vi "Get minimum separation within sphere.vi"(0 "Triangles to test":T2[](array[typedef]), 1 "Query triangles":T2[](array[typedef]), 2 "Octree for query triangles":T3[](array[typedef]), 3 "Sphere of interest":T1) -> (6 "Minimum separation vector\n(from all test triangles)":sgl[](array[numeric]), 7 "Minimum separation":sgl, 8 "Indices of possible triangles":i32[](array[numeric]))   [LabVIEW 2017]
doc: "This VI returns all the collision points between the test triangle and the query triangles, as well as the minimum separation vector and distance in the case of no collision."
uses:
  Typedefs/Triangle.ctl
  Typedefs/TreeNodeBox.ctl
  Typedefs/Quad.ctl
  Typedefs/Quadplane enum.ctl
  Typedefs/Sphere.ctl
panel:
  # "PN 13/03/2015"
  # "Vertices"
  # "Edges"
  # "Unit normal"
  # "Edge unit normals"
  # "Vertices"
  # "Edges"
  # "Unit normal"
  # "Plane ident."
  # "Vertices"
  # "Edges"
  # "Unit normal"
  # "Plane ident."
  # "Vertices"
  # "Edges"
  # "Unit normal"
  # "Plane ident."
  # "Vertices"
  # "Edges"
  # "Unit normal"
  # "Plane ident."
  # "Vertices"
  # "Edges"
  # "Unit normal"
  # "Plane ident."
  # "Vertices"
  # "Edges"
  # "Unit normal"
  # "Plane ident."
  # "Vertices"
  # "Edges"
  # "Unit normal"
  # "Edge unit normals"
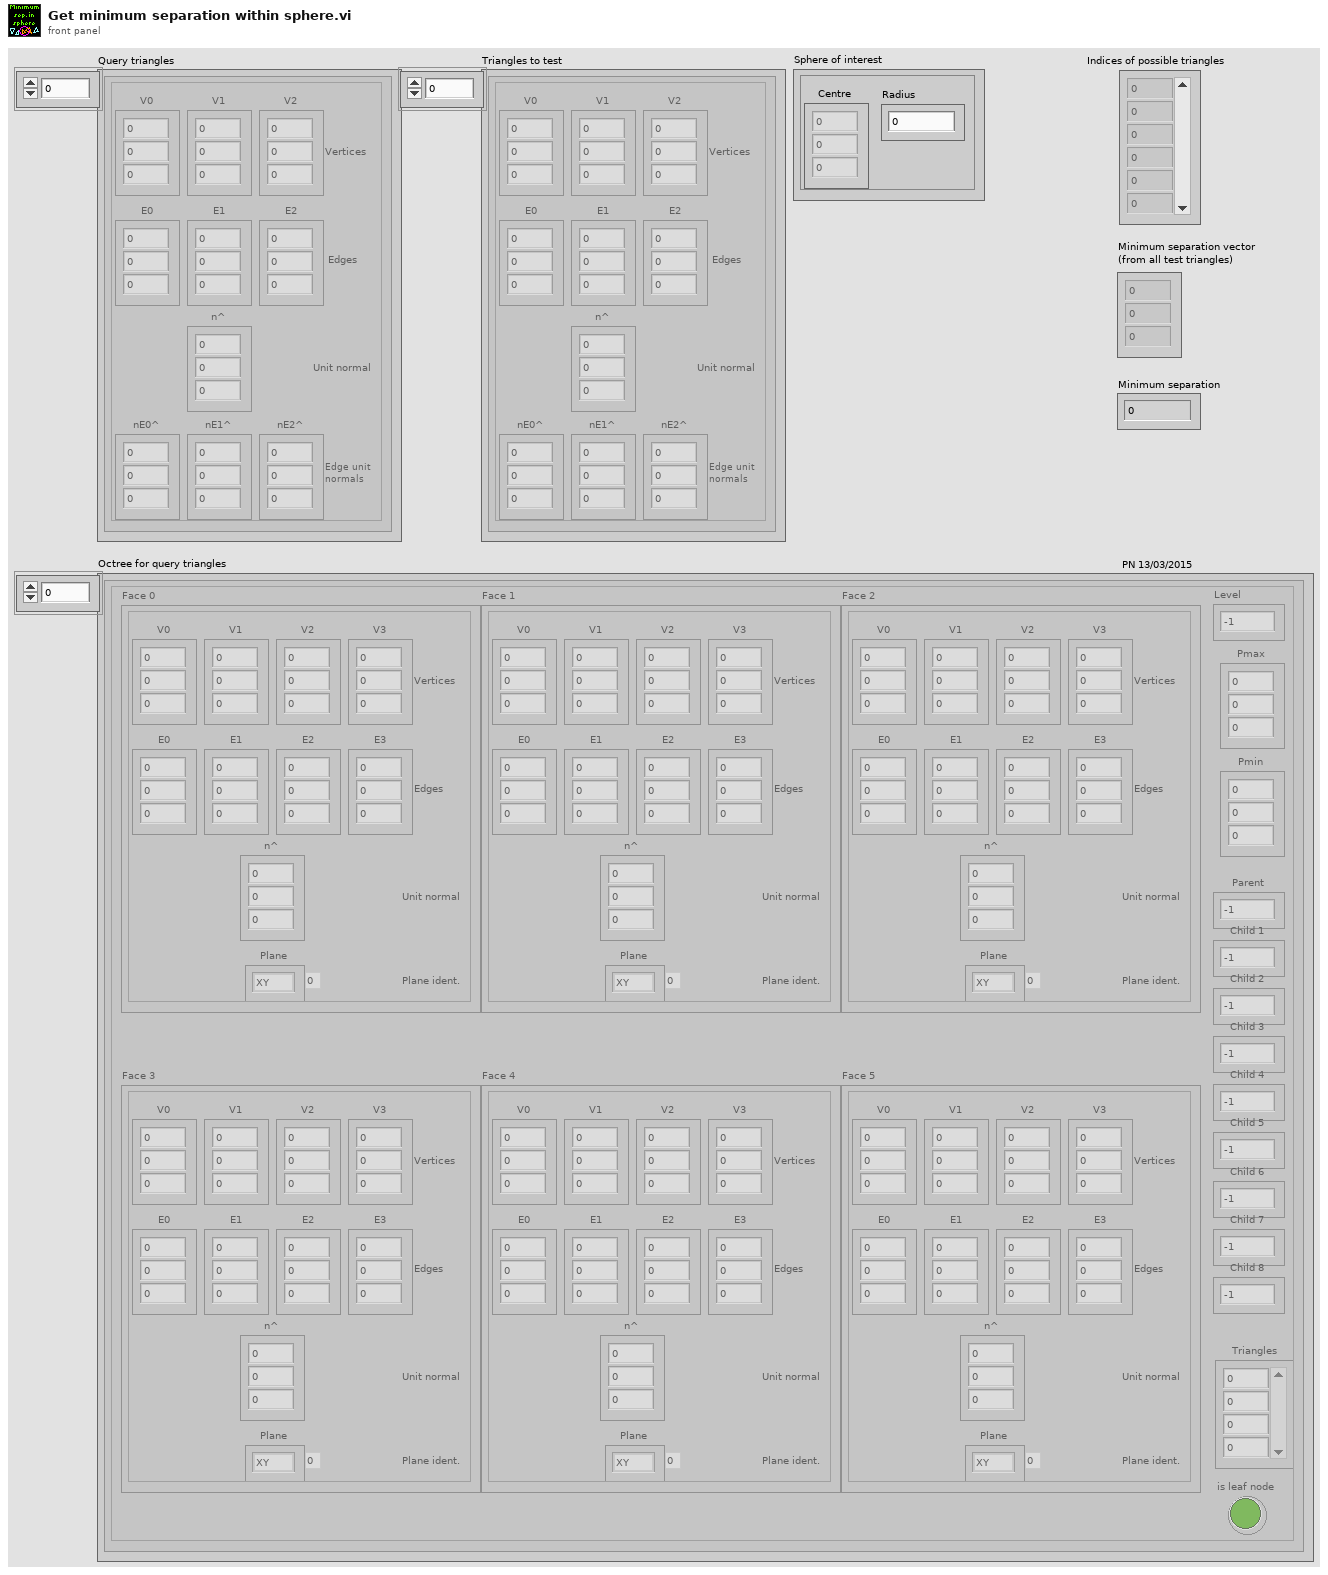
[diagram p1: front panel]
types:
  T1 = typedef "Sphere.ctl" = cluster{"Centre":sgl[], "Radius":sgl}
  T2 = typedef "Triangle.ctl" = cluster{"V0":sgl[], "V1":sgl[], "V2":sgl[], "E0":sgl[], "E1":sgl[], "E2":sgl[], "n^":sgl[], "nE0^":sgl[], "nE1^":sgl[], "nE2^":sgl[]}
  T3 = typedef "TreeNodeBox.ctl" = cluster{"Face 0":T4, "Face 1":T4, "Face 2":T4, "Face 3":T4, "Face 4":T4, "Face 5":T4, "Level":i32, "Pmax":sgl[], "Pmin":sgl[], "Parent":i32, "Child 1":i32, "Child 2":i32, "Child 3":i32, "Child 4":i32, "Child 5":i32, "Child 6":i32, "Child 7":i32, "Child 8":i32, "Triangles":i32[], "is leaf node":bool}
  T4 = typedef "Quad.ctl" = cluster{"V0":sgl[], "V1":sgl[], "V2":sgl[], "V3":sgl[], "E0":sgl[], "E1":sgl[], "E2":sgl[], "E3":sgl[], "n^":sgl[], "Plane":T5}
  T5 = typedef "Quadplane enum.ctl" = enum8{"XY", "XZ", "YZ", "-XY", "-XZ", "-YZ"}
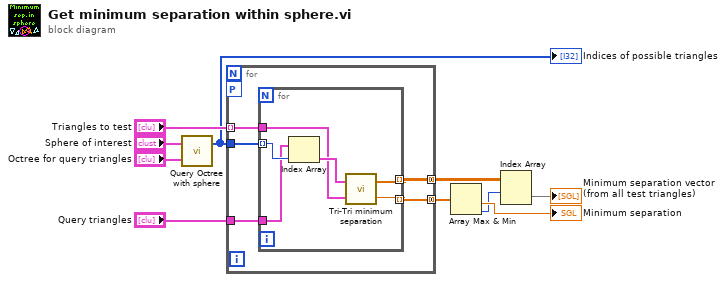
[diagram p0: block diagram]
diagram:
  n1 = call "Query Octree with sphere.vi"("Octree node array"="Octree for query triangles", "Sphere"="Sphere of interest") -> ("Indices of possible triangles"=w2:i32[])  [unwired: 1 out]
  "Indices of possible triangles" <- w2
  n2 = for {
    tunnel: [w15] -> w9 mode=concatenating
    tunnel: "Triangles to test" -> [w14] mode=indexing
    tunnel: [w13] -> w3 mode=concatenating
    tunnel: w2 -> [w12]
    tunnel: "Query triangles" -> [w11]
    workers-P: _ -> [_]
    n3 = for {
      tunnel: w14 -> [w18]
      tunnel: w12 -> [w21] mode=indexing
      tunnel: [w20] -> w15 mode=indexing
      tunnel: [w17] -> w13 mode=indexing
      tunnel: w11 -> [w16]
      n4 = Index Array(array=w16, index=w21) -> (element=w19:T2)
      n5 = call "Tri-Tri minimum separation.vi"("Triangle 2"=w18, "Triangle 1"=w19) -> ("Minimum separation distance"=w20:sgl, "Minimum separation vector\nfrom triangle 2 to triange 1"=w17:sgl[])
    }
  }
  n6 = Array Max & Min(array=w9) -> (min value=→"Minimum separation":sgl, min index (indices)=w4:i32)  [unwired: 2 out]
  n7 = Index Array(array=w3, index (row)=w4) -> (element=→"Minimum separation vector\n(from all test triangles)":sgl[])  [unwired: 1 in]
